vi "initialise.vi"(0 "VISA resource name":refnum<visa-resource-name>, 11 "error in (no error)":errorcluster) -> (4 "VISA resource name out":refnum<visa-resource-name>, 12 "Cold Head Temperature / K":dbl format="%.4f", 14 "Current Setpoint / K":dbl format="%.5f", 15 "error out":errorcluster)   [LabVIEW 2023]
uses:
  <instrlib>/Lake Shore 336/Public/Data/Sensor Data (Single Reading).vi
  <instrlib>/Lake Shore 336/Lake Shore 336.lvlib
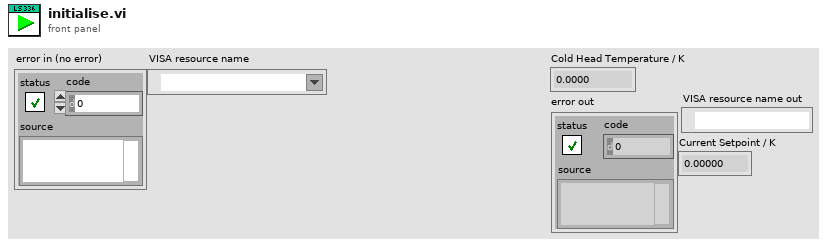
[diagram p1: front panel]
types:
  T1 = cluster{"Baud Rate":u32, "Parity":u16, "Data Bits":u16, "Stop Bits":u16, "Flow Control":u16}
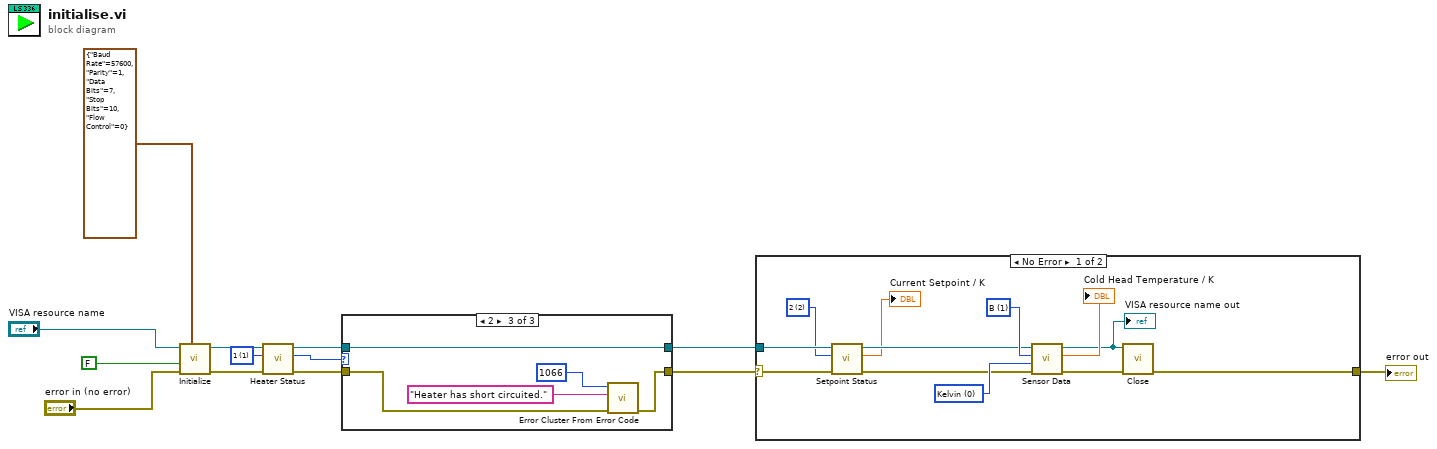
[diagram p0: block diagram]
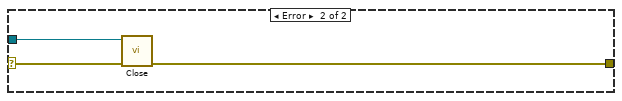
[diagram p2: hidden frame]
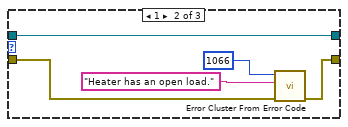
[diagram p4: hidden frame]
diagram:
  w7 = u16 1 items=["1"=1, "2"=2] ("Heater Output (1:1)")
  n1 = call <instrlib>:"Initialize.vi"("Serial Configuration"=T1 {"Baud Rate"=57600, "Parity"=1, "Data Bits"=7, "Stop Bits"=10, "Flow Control"=0}, "error in (no error)"="error in (no error)", "Reset (True)"=FALSE, "VISA resource name"="VISA resource name") -> ("error out"=w8:errorcluster, "VISA resource name out"=w9:refnum<visa-resource-name>)  [unwired: 6 in]
  n2 = call <instrlib>:"Heater Status.vi"("error in (no error)"=w8, "Heater Output (1:1)"=w7, "VISA resource name"=w9) -> ("error out"=w4:errorcluster, "Heater Status"=w6:u16, "VISA resource name out"=w5:refnum<visa-resource-name>)  [unwired: 6 in]
  n3 = case shown="2" w6 {
    tunnel: w5 -> [w15 w19 w24]
    tunnel: w4 -> [w14 w20 w25]
    tunnel: [w15 w19 w24] -> w3
    tunnel: [w14 w18 w23] -> w2
    frame 0, Default {
    }
    frame 1 {
      n4 = call <vilib>:"Error Cluster From Error Code.vi"("error in (no error)"=w20, "error message (\"\")"="Heater has an open load." ("error message (\"\")"), "error code (0)"=1066) -> ("error out"=w18:errorcluster)  [unwired: 6 in]
    }
    frame 2 {
      n5 = call <vilib>:"Error Cluster From Error Code.vi"("error in (no error)"=w25, "error message (\"\")"="Heater has short circuited." ("error message (\"\")"), "error code (0)"=1066) -> ("error out"=w23:errorcluster)  [unwired: 6 in]
    }
  }
  n6 = case shown="No Error" w2 {
    selector: w2 -> [w27 w39]
    tunnel: w3 -> [w37 w40]
    tunnel: [w26 w38] -> w1
    frame No Error {
      w29 = u16 2 items=["1"=1, "2"=2, "3"=3, "4"=4] ("Output (1:1)")
      w33 = u16 0 items=["Kelvin", "Celsius", "Sensor Units"] ("Data Source (0:Kelvin)")
      w36 = u16 1 items=["A", "B", "C", "D"] ("Input (0:A)")
      n7 = call <instrlib>:"Setpoint Status.vi"("error in (no error)"=w27, "Output (1:1)"=w29, "VISA resource name"=w37) -> ("error out"=w30:errorcluster, "Setpoint"=→"Current Setpoint / K":dbl, "VISA resource name out"=w31:refnum<visa-resource-name>)  [unwired: 6 in]
      n8 = call-poly <instrlib>:"Sensor Data.vi"("error in (no error)"=w30, "Data Source (0:Kelvin)"=w33, "Input (0:A)"=w36, "VISA resource name"=w31) -> ("error out"=w32:errorcluster, "Sensor Data"=→"Cold Head Temperature / K":dbl, "VISA resource name out"=w34:refnum<visa-resource-name>)  [unwired: 5 in]
      "VISA resource name out" <- w34
      n9 = call <instrlib>:"Close.vi"("error in (no error)"=w32, "VISA resource name"=w34) -> ("error out"=w26:errorcluster)  [unwired: 9 in]
    }
    frame Error {
      n10 = call <instrlib>:"Close.vi"("error in (no error)"=w39, "VISA resource name"=w40) -> ("error out"=w38:errorcluster)  [unwired: 9 in]
    }
  }
  "error out" <- w1
